vi "AssertConnectorPanesMatchExpected.vi"(8 "error in (no error)":errorcluster, 10 "custom device xml path":path, 11 "TestCase in":refnum<class "TestCase.lvclass">) -> (0 "error out":errorcluster, 3 "TestCase out":refnum<class "TestCase.lvclass">)   [LabVIEW 2015, in "VeriStandTestUtilities.lvlib"]
uses:
  VeriStandTestUtilities.lvlib
  <vilib>/addons/_JKI Toolkits/VI Tester/TestCase.llb/TestCase.lvclass
  ConnectorPaneTemplate.ctl
  <vilib>/NI Veristand/Custom Device API/Custom Device Execution Mode.ctl
  <userlib>/_OpenG.lib/file/file.llb/Append Path to Root if Relative - Scalar__ogtk.vi
  <vilib>/NI VeriStand/Custom Device API/Custom Device API.lvlib
panel:
  in  "connector pane templates":T1[](array[typedef])=[{"Template File"=path "NI Veristand/Custom Device API/ActionVIOnCompile Template.vit", "XPath Key"="//ActionVIOnCompile/Path/text()"}, {"Template File"=path "NI Veristand/Custom Device API/ActionVIOnDelete Template.vit", "XPath Key"="//ActionVIOnDelete/Path/text()"}, {"Template File"=path "NI Veristand/Custom Device API/ActionVIOnDeleteRequest Template.vit", "XPath Key"="//ActionVIOnDeleteRequest/Path/text()"}, {"Template File"=path "NI Veristand/Custom Device API/ActionVIOnDownload.vit", "XPath Key"="//ActionVIOnDownload/Path/text()"}, {"Template File"=path "NI Veristand/Custom Device API/ActionVIOnLoad Template.vit", "XPath Key"="//ActionVIOnLoad/Path/text()"}, {"Template File"=path "NI Veristand/Custom Device API/ActionVIOnPaste Template.vit", "XPath Key"="//ActionVIOnPaste/Path/text()"}, {"Template File"=path "NI Veristand/Custom Device API/ActionVIOnSave Template.vit", "XPath Key"="//ActionVIOnSave/Path/text()"}, {"Template File"=path "NI Veristand/Custom Device API/ActionVIOnShutdown Template.vit", "XPath Key"="//ActionVIOnSystemShutdown/Path/text()"}, {"Template File"=path "NI Veristand/Custom Device API/Page Template.vit", "XPath Key"="//Page/Item2Launch/Path/text()"}, {"Template File"=path "NI Veristand/Custom Device API/Initialization VI Template.vit", "XPath Key"="//InitializationVI/Item2Launch/Path/text()"}, {"Template File"=path "NI Veristand/Custom Device API/RunTimeMenu Custom Item 2 Launch.vit", "XPath Key"="//RunTimeMenu/MenuItem[Type=\"Action\"]/Item2Launch/Path/text()"}, {"Template File"=path "NI Veristand/Custom Device API/Timing Source Initialization VI Template.vit", "XPath Key"="//TimingSource//RealTimeSystemDestination/text()"}]
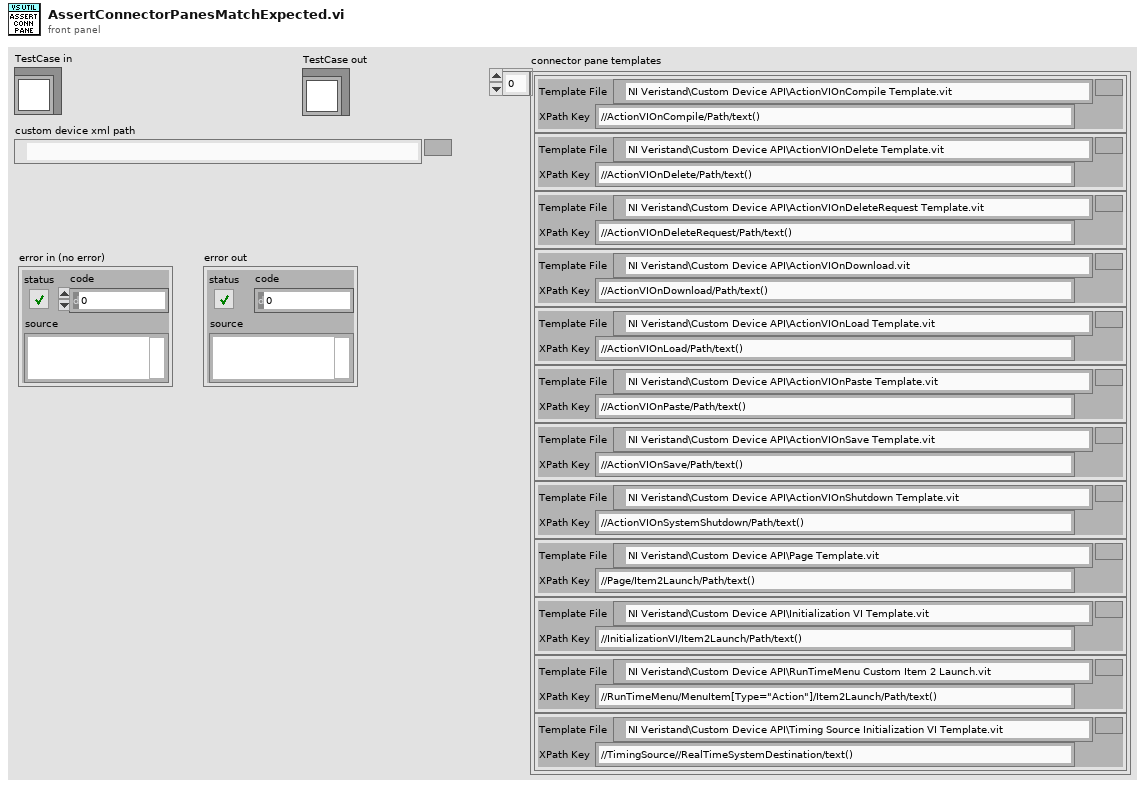
[diagram p1: front panel]
types:
  T1 = typedef "VeriStandTestUtilities.lvlib/ConnectorPaneTemplate.ctl" = cluster{"Template File":path, "XPath Key":string}
  T2 = typedef "Custom Device API.lvlib/Custom Device Execution Mode.ctl" = enum16{"Asynchronous", "Inline HW Interface", "Inline Model Interface", "Inline Timing and Sync", "Asynchronous Timing and Sync"}
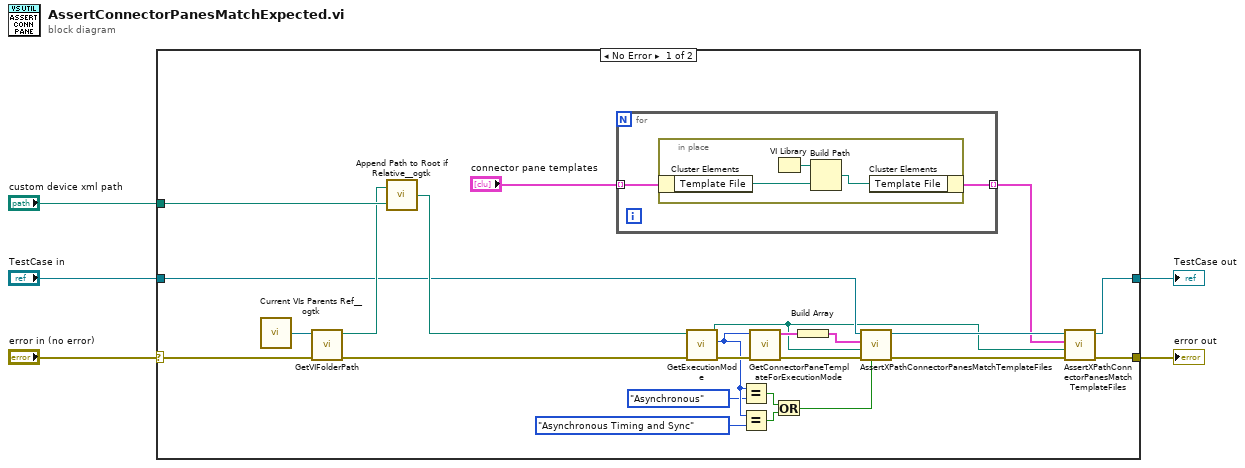
[diagram p0: block diagram]
diagram:
  n1 = case shown="No Error" "error in (no error)" {
    selector: "error in (no error)" -> [w22 w36]
    tunnel: [w28 w36] -> w5
    tunnel: "custom device xml path" -> [w29 _]
    tunnel: "TestCase in" -> [w16 w35]
    tunnel: [w27 w35] -> w1
    frame No Error {
      n2 = call <userlib>:"Current VIs Parents Ref__ogtk.vi"() -> ("Calling VI's Reference"=w24:refnum<vi>)  [unwired: 2 in]
      n3 = call "GetVIFolderPath.vi"("error in (no error)"=w22, "VI Reference in"=w24) -> ("error out"=w23:errorcluster, "VI Folder Path out"=w21:path)  [unwired: 8 in]
      n4 = call-poly <userlib>:"Append Path to Root if Relative__ogtk.vi"("Absolute or Relative Path"=w29, "Root Path"=w21) -> ("Absolute or Appended Path"=w25:path)
      n5 = for {
        tunnel: "connector pane templates" -> [w31] mode=indexing
        tunnel: [w30] -> w14 mode=indexing
        n6 = in-place {
          n7 = in-place-cluster #1(w31) -> ("Template File"=w32:path)
          n8 = VI Library() -> (path=w34:path)
          n9 = Build Path(base path=w34, name or relative path=w32) -> (appended path=w33:path)
          n10 = in-place-cluster #1("Template File"=w33) -> (w30:T1)
        }
      }
      n11 = call "GetExecutionMode.vi"("error in (no error)"=w23, "absolute custom device xml file"=w25) -> ("error out"=w20:errorcluster, "execution mode"=w8:T2, "absolute custom device xml file"=w9:path)  [unwired: 7 in]
      n12 = Equal?(x=w8, y=Custom_Device_Execution_Mode."Asynchronous") -> (x = y?=w11:bool)
      n13 = Equal?(x=w8, y=Custom_Device_Execution_Mode."Asynchronous Timing and Sync") -> (x = y?=w12:bool)
      n14 = call "GetConnectorPaneTemplateForExecutionMode.vi"("error in (no error)"=w20, "execution mode"=w8) -> ("error out"=w18:errorcluster, "connector pane template"=w19:T1)  [unwired: 8 in]
      n15 = Or(x=w11, y=w12) -> (x .or. y?=w10:bool)
      n16 = Build Array(w19) -> (w17:T1[])
      n17 = call "AssertXPathConnectorPanesMatchTemplateFiles.vi"("terminal subset acceptable (false)"=w10, "error in (no error)"=w18, "absolute custom device xml file"=w9, "connector pane templates"=w17, "TestCase in"=w16) -> ("error out"=w13:errorcluster, "TestCase out"=w15:refnum<class "TestCase.lvclass">)  [unwired: 5 in]
      n18 = call "AssertXPathConnectorPanesMatchTemplateFiles.vi"("error in (no error)"=w13, "absolute custom device xml file"=w9, "connector pane templates"=w14, "TestCase in"=w15) -> ("error out"=w28:errorcluster, "TestCase out"=w27:refnum<class "TestCase.lvclass">)  [unwired: 6 in]
    }
    frame Error {
    }
  }
  "error out" <- w5
  "TestCase out" <- w1
